vi "Nimbelink_Database_Check_For_Duplicates polaris.vi"(6 "Error in (no error)":errorcluster, 9 "Work order":string) -> (0 "Error out":errorcluster, 1 "Distinct Passed Units Cnt":i32, 2 "Duplicate serial numbers":string[](array[string]), 3 "Duplicate serial numbers?":bool, 4 "PostTestPasses":i32, 5 "PreTestPasses":i32)   [LabVIEW 2013]
uses:
  Test Globals/Global 1.vi
panel:
  out "RecordSet 2":string[][](array[string])
  out "RecordSet":string[][](array[string])
  in  "ConnectionString":string="Provider=SQLOLEDB.1;User Id=SSTest;Password=test;Initial Catalog=Nimbelink;Data Source=BTWSQLSVR\\TESTDEPT "
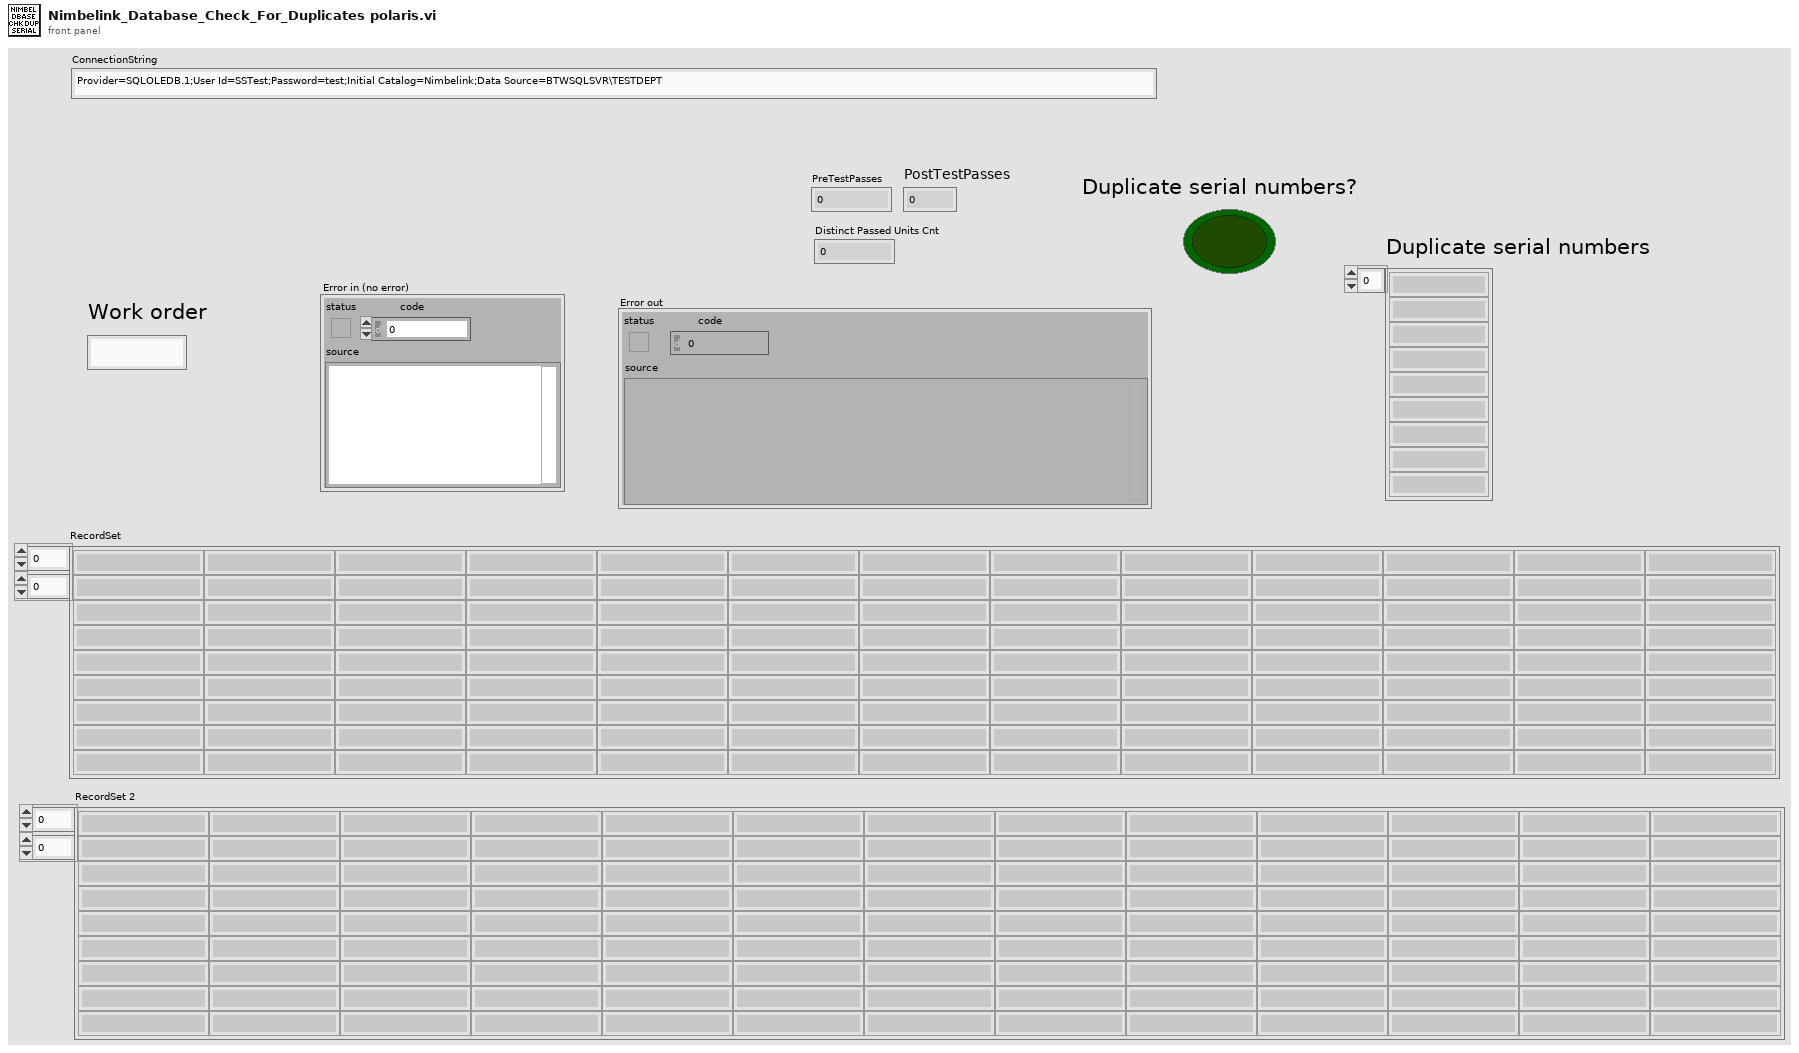
[diagram p1: front panel]
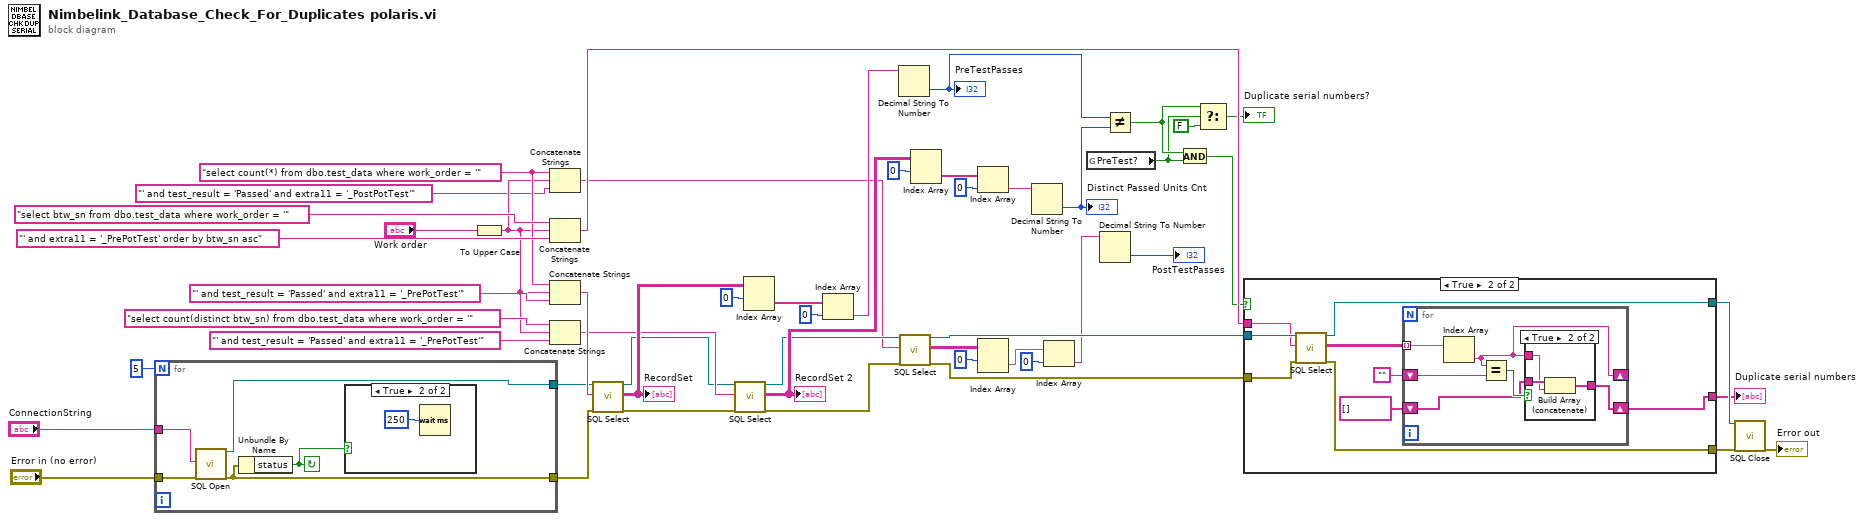
[diagram p0: block diagram]
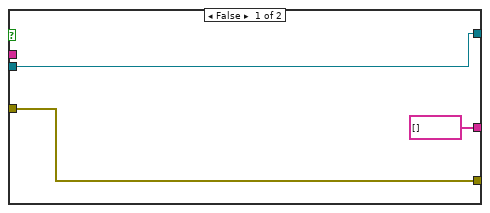
[diagram p2: hidden frame]
diagram:
  w10 = "select count(*) from dbo.test_data where work_order = '" ("string")
  n1 = for {
    N: 5 -> [_]
    tunnel: "ConnectionString" -> [w56]
    tunnel: "Error in (no error)" -> [w55]
    tunnel: [w54] -> w40
    tunnel: [w53] -> w44
    stop <- w52 continue-if-true
    n2 = call "SQL Open.vi"("ConnectionString In"=w56, "Error in (no error)"=w55) -> ("Connection Out"=w54:refnum<k7>, "Error out"=w53:errorcluster)  [unwired: 16 in]
    n3 = Unbundle By Name(w53) -> ("status"=w52:bool)
    n4 = case shown="True" w52 {
      frame False {
      }
      frame True {
        n5 = Wait (ms)(milliseconds to wait=u32 250) -> ()  [unwired: 1 out]
      }
    }
  }
  n6 = To Upper Case(1:"Work order") -> (0:w9:string)
  n7 = Concatenate Strings(w10, w9, "' and test_result = 'Passed' and extra11 = '_PostPotTest'" ("string")) -> (w11:string)
  n8 = Concatenate Strings("select btw_sn from dbo.test_data where work_order = '" ("string"), w9, "' and extra11 = '_PrePotTest' order by btw_sn asc" ("string")) -> (w21:string)
  n9 = Concatenate Strings(w10, w9, "' and test_result = 'Passed' and extra11 = '_PrePotTest'" ("string")) -> (w42:string)
  n10 = Concatenate Strings("select count(distinct btw_sn) from dbo.test_data where work_order = '" ("string"), w9, "' and test_result = 'Passed' and extra11 = '_PrePotTest'" ("string")) -> (w32:string)
  n11 = call "SQL Select.vi"("Connection In"=w40, "SQL Query"=w42, "Error in (no error)"=w44) -> ("Connection Out"=w30:refnum<k7>, "Data"=w45:string[][], "Error out"=w31:errorcluster)  [unwired: 14 in]
  "RecordSet" <- w45
  n12 = call "SQL Select.vi"("Connection In"=w30, "SQL Query"=w32, "Error in (no error)"=w31) -> ("Connection Out"=w13:refnum<k7>, "Data"=w39:string[][], "Error out"=w14:errorcluster)  [unwired: 14 in]
  "RecordSet 2" <- w39
  n13 = Index Array(array=w45, index (row)=0) -> (element=w47:string[])  [unwired: 1 in]
  n14 = Index Array(array=w47, index=0) -> (element=w49:string)
  n15 = Decimal String To Number(string=w49) -> (number=w27:i32)  [unwired: 2 in, 1 out]
  "PreTestPasses" <- w27
  n16 = call "SQL Select.vi"("Connection In"=w13, "SQL Query"=w11, "Error in (no error)"=w14) -> ("Connection Out"=w12:refnum<k7>, "Data"=w4:string[][], "Error out"=w1:errorcluster)  [unwired: 14 in]
  n17 = Index Array(array=w39, index (row)=0) -> (element=w37:string[])  [unwired: 1 in]
  n18 = Index Array(array=w37, index=0) -> (element=w35:string)
  n19 = Index Array(array=w4, index (row)=0) -> (element=w3:string[])  [unwired: 1 in]
  n20 = Decimal String To Number(string=w35) -> (number=w26:i32)  [unwired: 2 in, 1 out]
  "Distinct Passed Units Cnt" <- w26
  n21 = Index Array(array=w3, index=0) -> (element=w6:string)
  n22 = global read "Global 1.vi" "PreTest?"() -> (w16:bool)
  n23 = Decimal String To Number(string=w6) -> (number=→"PostTestPasses":i32)  [unwired: 2 in, 1 out]
  n24 = Not Equal?(x=w27, y=w26) -> (x != y?=w17:bool)
  n25 = And(x=w17, y=w16) -> (x .and. y?=w15:bool)
  n26 = Select(t=w17, s=w16, f=FALSE) -> (s? t:f=→"Duplicate serial numbers?":bool)
  n27 = case shown="True" w15 {
    tunnel: w12 -> [w60 w69]
    tunnel: [w58 w62] -> w25
    tunnel: [w60 w63] -> w24
    tunnel: w21 -> [_ w68]
    tunnel: [string[] [] w64] -> w20
    tunnel: w1 -> [w58 w61]
    frame False {
    }
    frame True {
      n28 = call "SQL Select.vi"("Connection In"=w69, "SQL Query"=w68, "Error in (no error)"=w61) -> ("Connection Out"=w63:refnum<k7>, "Data"=w67:string[][], "Error out"=w62:errorcluster)  [unwired: 14 in]
      n29 = for {
        tunnel: w67 -> [w75] mode=indexing
        shift-right: [w70] -> _
        shift-left: "" -> [w74]
        shift-right: [w71] -> w64
        shift-left: string[] [] -> [w72]
        n30 = Index Array(array=w75) -> (element=w70:string)  [unwired: 1 in]
        n31 = Equal?(x=w70, y=w74) -> (x = y?=w73:bool)
        n32 = case shown="True" w73 {
          tunnel: w72 -> [w76 w79]
          tunnel: w70 -> [_ w78]
          tunnel: [w76 w77] -> w71
          frame False {
          }
          frame True {
            n33 = Build Array (concatenate)(w79, w78) -> (w77:string[])
          }
        }
      }
    }
  }
  "Duplicate serial numbers" <- w20
  n34 = call "SQL Close.vi"("Connection In"=w24, "Error in (no error)"=w25) -> ("Error out"=→"Error out":errorcluster)  [unwired: 17 in]
